vi "Ultrasonic_range_finder2.vi"(0 "FPGA I/O Out (Trigger Pulse)":refnum<k21>="ConnectorC/DIO4", 2 "Control On/Off":bool, 5 "FPGA I/O In (Echo)":refnum<k21>="ConnectorC/DIO1", 7 "FPGA I/O In (Control On/Off)":refnum<k21>="Pump_Control", 9 "Low Pulse (usec)":u32=100000, 11 "High Pulse(usec)":u32=5) -> (4 "Output Pulse":bool, 6 "Measured Period (usec)":u32)   [LabVIEW 2013]
doc: "Function #1: This VI generates a pulse width modulated output with programmable \nhigh and low periods to act as a trigger pulse for the Parallax Ping ))) sensor.\n\nFunction#2: This VI measures the pulsewidth of the received echo and converts it to distance (inch or cm).\n\nFunction#3: Based on the calculation done in the host VI, once a certain distance is reached the VI turns the \ncontrolled device (e.g. pump or heater) On/Off"
uses:
  <vilib>/Platform/TimedLoop/XDataNode/timing_clust.ctl
  <vilib>/Platform/TimedLoop/XDataNode/nitl_modes.ctl
  <vilib>/Platform/TimedLoop/XDataNode/wakeup.ctl
  <vilib>/rvi/Emulation/niFpgaSctlEmulationGetInTimedLoop.vi
  <vilib>/rvi/Emulation/niFpgaEmulationReportErrorSimple.vi
  <vilib>/rvi/Emulation/niFpgaGetClockAttributes.vi
  Instance           1 23Saved   PWM Out, Simple .vi
  <vilib>/rvi/eio/common/nirviEmuTemplateMethod_errors.vi
  <vilib>/rvi/Emulation/niFpgaCriticalErrorInLSC.vi
  <vilib>/Platform/TimedLoop/XDataNode/XDataNode.xnode
  <vilib>/eio/EIONode/EIONode.xnode
  <vilib>/Platform/TimedLoop/XDataNode/XDNodeRunTimeDep.lvlib
panel:
  in  "stop 3":bool
  in  "Pulsewidth Polarity":bool
  in  "stop 2":bool
  out "Input Signal (Out)":bool
  in  "stop":bool
  # "Function #1: This VI generates a pulse width modulated output with programmable \nhigh and low periods to act as a trigger pulse for the Parallax Ping ))) sensor.\n\nFunction#2: This VI measures the pulsewidth of the received echo and converts it to distance (inch or cm).\n\nFunction#3: Based on the calculation done in the host VI, once a certain distance is reached the VI turns the \ncontrolled device (e.g. pump or heater) On/Off"
  # "100ms"
  # "5usec"
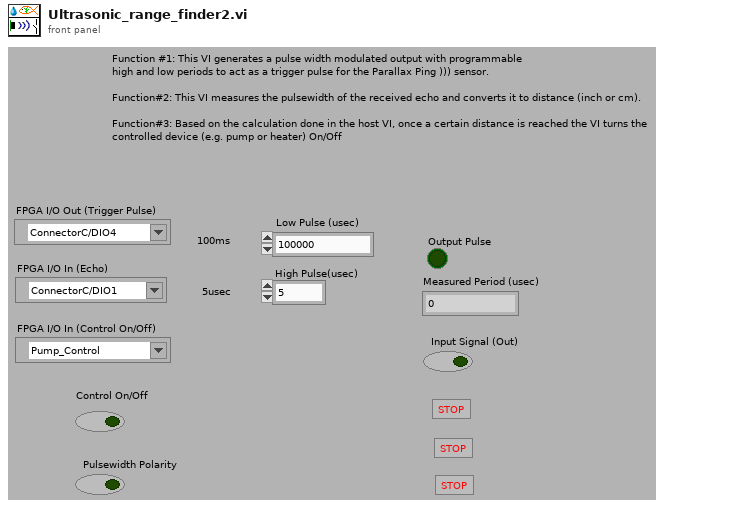
[diagram p1: front panel]
types:
  T1 = typedef "XDNodeRunTimeDep.lvlib/timing_clust.ctl" = cluster{"Expected End [f-1]":u64, "Actual End [f-1]":u64, "Finished Late? [f-1]":bool, "Expected End [i-1]":u64, "Actual End [i-1]":u64, "Finished Late? [i-1]":bool, "Expected Start [i]":u64, "Actual Start [i]":u64, "Expected Start [f]":u64, "Actual Start [f]":u64, "Source Name":string, "Structure Name":string, "Period":i64, "Deadline":i64, "Offset":i64, "Start":i64, "Priority":i32, "Timeout":i32, "Mode":T2, "Wakeup Reason":T3, "Error":errorcluster, "Source Type":string, "Secondary Source Type":string, "Global End Time":u64, "Global Start Time":u64, "Frame Duration":u64, "Iteration Duration":u64, "Assigned CPU":i32, "I/O Scan Engine Mode":u32}
  T2 = typedef "XDNodeRunTimeDep.lvlib/nitl_modes.ctl" = enum32{"No Change", "Process missed periods, maintain original phase", "Discard missed periods, maintain original phase", "Process missed periods, ignore original phase", "Discard missed periods, ignore original phase"}
  T3 = typedef "XDNodeRunTimeDep.lvlib/wakeup.ctl" = enum32{"Normal", "Aborted", "Asynchronous wakeup", "Timing source error", "Timed loop error", "Timeout"}
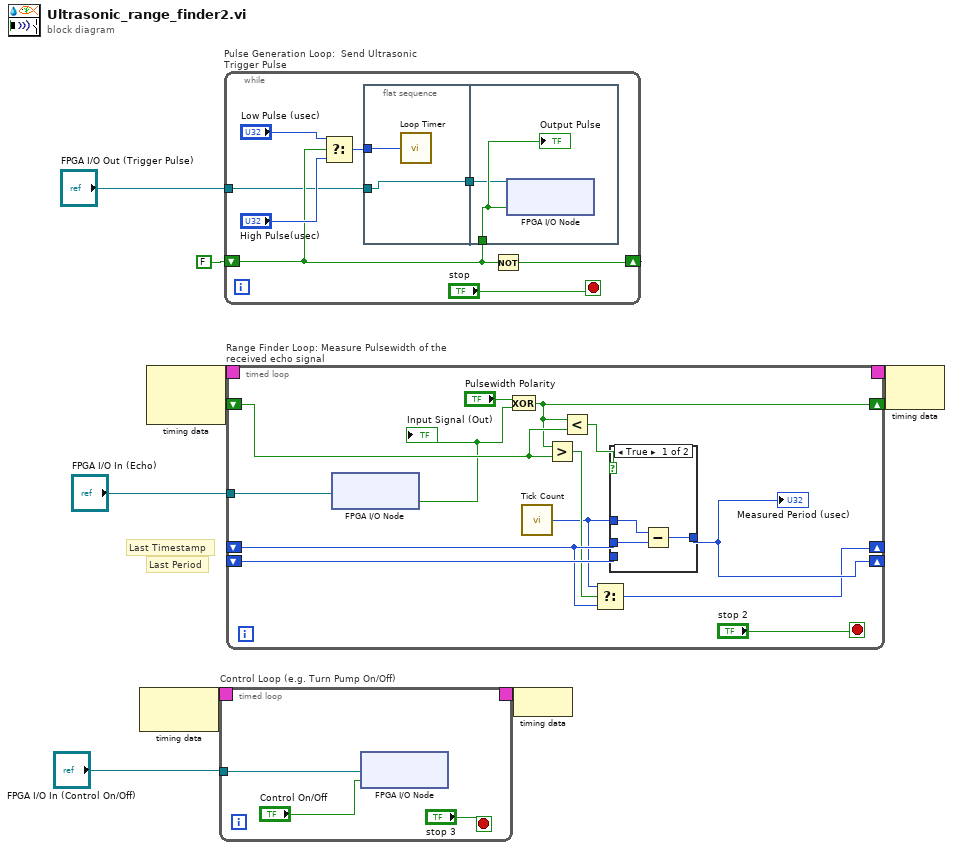
[diagram p0: block diagram]
diagram:
  # "Last Period"
  # "Last Timestamp"
  n1 = node-c288() -> (w3:T1)  [unwired: 1 in]
  n2 = node-c288() -> (w7:T1)  [unwired: 2 out]
  n3 = timed-loop "Control Loop (e.g. Turn Pump On/Off)" {
    timing: w3 -> [_]
    timing-out: [_] -> w2
    tunnel: "FPGA I/O In (Control On/Off)" -> [w10]
    stop <- "stop 3" stop-if-true
    n4 = xnode "FPGA I/O Node"("I/O Item"="Control On/Off", "FPGA I/O In"=w10) -> ()  [unwired: 1 out]
  }
  n5 = while "Pulse Generation Loop:  Send Ultrasonic Trigger Pulse" {
    shift-right: [w17] -> _
    shift-left: FALSE -> [w18]
    tunnel: "FPGA I/O Out (Trigger Pulse)" -> [w15]
    stop <- "stop" stop-if-true
    n6 = Select(t="Low Pulse (usec)", s=w18, f="High Pulse(usec)") -> (s? t:f=w19:u32)
    n7 = flat-sequence {
      tunnel: w19 -> [w23]
      tunnel: w15 -> [w22]
      tunnel: [w22] -> w14
      tunnel: w18 -> [w25]
      tunnel: w14 -> [w24]
      frame #0 {
        n8 = call "Loop Timer"("Count(uSec)"=w23) -> ()  [unwired: 1 out]
      }
      frame #1 {
        n9 = xnode "FPGA I/O Node"("I/O Item"=w25, "FPGA I/O In"=w24) -> ()  [unwired: 1 out]
        "Output Pulse" <- w25
      }
    }
    n10 = Not(x=w18) -> (.not. x?=w17:bool)
  }
  n11 = timed-loop "Range Finder Loop: Measure Pulsewidth of the received echo signal" {
    timing-out: [_] -> w6
    timing: w7 -> [_]
    shift-left: _ -> [w36]
    shift-right: [w37] -> _
    shift-left: _ -> [w35]
    shift-right: [w34] -> _
    shift-left: _ -> [w32]
    shift-right: [w30] -> _
    tunnel: "FPGA I/O In (Echo)" -> [w26]
    stop <- "stop 2" stop-if-true
    n12 = xnode "FPGA I/O Node"("FPGA I/O In"=w26) -> ("I/O Item"=w27:bool)  [unwired: 1 out]
    "Input Signal (Out)" <- w27
    n13 = Exclusive Or(1:w27, 2:"Pulsewidth Polarity") -> (0:w30:bool)
    n14 = call "Tick Count"() -> ("Tick Count(uSec)"=w29:u32)
    n15 = Greater?(x=w30, y=w32) -> (0:w33:bool)
    n16 = Less?(x=w30, y=w32) -> (x < y?=w31:bool)
    n17 = Select(t=w29, s=w33, f=w35) -> (s? t:f=w34:u32)
    n18 = case shown="True" w31 {
      tunnel: w36 -> [_ w42]
      tunnel: w29 -> [w39 _]
      tunnel: w35 -> [w40 _]
      tunnel: [w41 w42] -> w37
      frame True {
        n19 = Subtract(x=w39, y=w40) -> (x-y=w41:u32)
      }
      frame False {
      }
    }
    "Measured Period (usec)" <- w37
  }
  n20 = node-c288(w2) -> ()
  n21 = node-c288(w6) -> ()  [unwired: 1 out]
